vi "Get Spectral Map (U8).vi"(6 "window info":T1={"window type"=10, "window length"=2048} {"window type" items=["None"=0, "Hanning"=1, "Hamming"=2, "Blackman-Harris"=3, "Exact Blackman"=4, "Blackman"=5, "Flat Top"=6, "4 Term B-Harris"=7, "7 Term B-Harris"=8, "Low Sidelobe"=9, "Gaussian"=62]; "window length" min=0}, 7 "dB On (T)":bool=TRUE, 8 "error in (no error)":errorcluster, 9 "type":T4(ring)=enum."RPM-Order", 10 "speed profile":T5 {"speed [RPM]" format="%.2f"; "time [s]" format="%.2f"}, 11 "scaled signal [EU]":waveform(dbl)={"t0"=timestamp(0 s since 1904-01-01), "dt"=0.0, "Y"=[]}) -> (0 "error out":errorcluster, 1 "unit labels":T2, 2 "scales":T3 {"Z scale"."multiplier" format="%.2f"; "Z scale"."offset" format="%.2f"; "Y scale"."multiplier" format="%.2f"; "Y scale"."offset" format="%.2f"; "X scale"."multiplier" format="%.2f"; "X scale"."offset" format="%.2f"}, 3 "spectral map":u8[][](array[numeric]), 4 "actual window":T1={"window type"=10, "window length"=2048} {"window type" items=["None"=0, "Hanning"=1, "Hamming"=2, "Blackman-Harris"=3, "Exact Blackman"=4, "Blackman"=5, "Flat Top"=6, "4 Term B-Harris"=7, "7 Term B-Harris"=8, "Low Sidelobe"=9, "Gaussian"=62]; "window length" min=0})   [LabVIEW 2017]
doc: "Returns the spectral map of <B>scaled signal [EU]</B>. You can use this polymorphic VI to return <B>spectral map</B> as a 2D array of double-precision, floating-point numbers or a 2D array of 8-bit unsigned integers. You must manually select the polymorphic instance to use. Use the DBL instance to obtain more accurate data. Use the U8 instance to reduce memory usage when the VI displays data."
uses:
  <vilib>/addons/Sound and Vibration/Order Analysis/Tach Process/SubVIs/speed profile.ctl
  <vilib>/addons/Sound and Vibration/Order Analysis/Ref Gabor Order Tracking/window information.ctl
  <vilib>/addons/Sound and Vibration/Order Analysis/Ref Gabor Order Tracking/Get Order-RPM Spectral Map (U8).vi
  <vilib>/addons/Sound and Vibration/Order Analysis/Ref Gabor Order Tracking/Get Freq-RPM Spectral Map (U8).vi
  <vilib>/addons/Sound and Vibration/Order Analysis/Ref Gabor Order Tracking/Get Freq-Time Spectral Map (U8).vi
  <vilib>/addons/_NISVFA/_Shared subVIs/Common/svc_Engineering Units to Unit Label.vi
  <vilib>/addons/_NISVFA/_Shared subVIs/Common/svc_Unit Label to Engineering Units.vi
  <vilib>/addons/Sound and Vibration/Order Analysis/Gabor Order Tracking/SoundVib_Gabor.lvlib
  <vilib>/addons/Sound and Vibration/Order Analysis/Tach Process/SoundVib_TachProcess.lvlib
panel:
  # "Get Spectral Map (U8)"
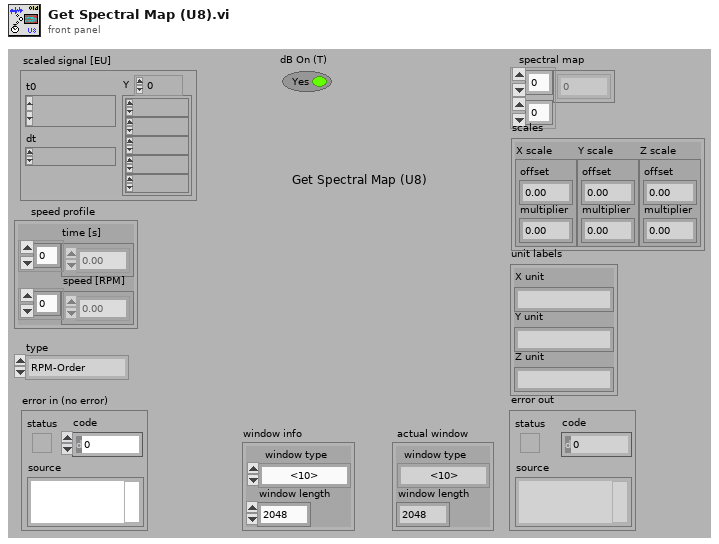
[diagram p1: front panel]
types:
  T1 = typedef "SoundVib_Gabor.lvlib/window information.ctl" = cluster{"window type":u32, "window length":i32}
  T2 = cluster{"X unit":string, "Y unit":string, "Z unit":string}
  T3 = cluster{"X scale":cluster{"offset":dbl, "multiplier":dbl}, "Y scale":cluster{"offset":dbl, "multiplier":dbl}, "Z scale":cluster{"offset":dbl, "multiplier":dbl}}
  T4 = enum16{"Frequency-Time", "Frequency-RPM", "Order-RPM", "RPM-Order"}
  T5 = typedef "SoundVib_TachProcess.lvlib/speed profile.ctl" = cluster{"time [s]":dbl[], "speed [RPM]":dbl[]}
  T6 = typedef "svc_Channel Info.ctl" = cluster{"sensor sensitivity":dbl, "engineering units":T7, "dB reference":dbl, "custom label":string, "weighting filter":T8, "pregain":dbl}
  T7 = typedef "svc_Engineering Units Text Ring.ctl" = u16
  T8 = typedef "svc_Weighting Filter Text Ring.ctl" = u16
  T9 = typedef "SoundVib_Gabor.lvlib/GT RefNum.ctl" = refnum<k1>
  T10 = cluster{"column unit":string, "row unit":string, "unit label":string}
  T11 = cluster{"order scale":cluster{"offset":dbl, "multiplier":dbl}, "rpm scale":cluster{"offset":dbl, "multiplier":dbl}, "quantization info":cluster{"offset":dbl, "multiplier":dbl}}
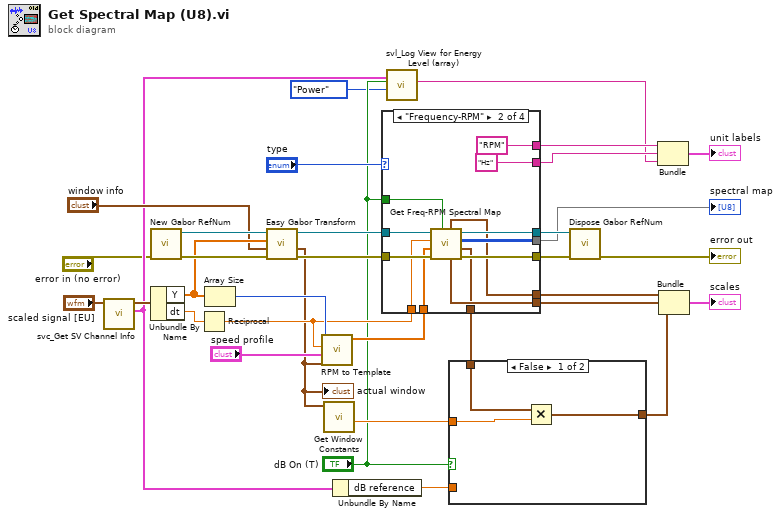
[diagram p0: block diagram]
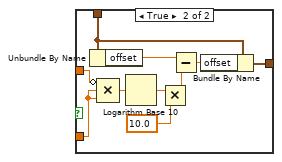
[diagram p2: hidden frame]
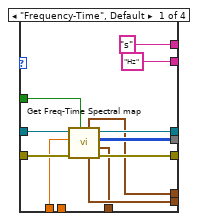
[diagram p3: hidden frame]
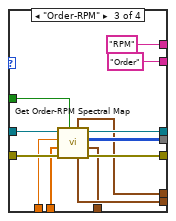
[diagram p4: hidden frame]
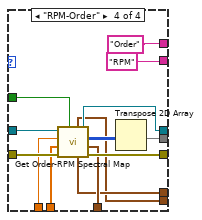
[diagram p5: hidden frame]
diagram:
  n1 = call <vilib>:"svc_Get SV Channel Info.vi"("scaled signal [EU]"="scaled signal [EU]") -> ("channel info"=w3:T6, "dup scaled signal [EU]"=w14:waveform(dbl))  [unwired: 5 in, 4 out]
  n2 = call <vilib>:"New Gabor RefNum.vi"("error in (no error)"="error in (no error)") -> ("error out"=w33:errorcluster, "RefNum"=w34:T9)  [unwired: 8 in]
  n3 = Unbundle By Name(w14) -> ("Y"=w21:dbl[], "dt"=w19:dbl)
  n4 = Reciprocal(x=w19) -> (1/x=w20:dbl)
  n5 = Array Size(array=w21) -> (size(s)=w27:i32)
  n6 = call <vilib>:"Easy Gabor Transform.vi"("error in (no error)"=w33, "window info"="window info", "x[n]"=w21, "RefNum in"=w34) -> ("error out"=w30:errorcluster, "actual window"=w8:T1, "RefNum out"=w31:T9)  [unwired: 3 in, 2 out]
  "actual window" <- w8
  n7 = call <vilib>:"RPM to Template.vi"("window info"=w8, "speed profile"="speed profile", "sampling frequency [Hz]"=w20, "signal length"=w27) -> ("Gabor template"=w25:dbl[])  [unwired: 6 in, 1 out]
  n8 = call <vilib>:"Get Window Constants.vi"("window info"=w8) -> ("multiply factor"=w7:dbl)  [unwired: 9 in, 1 out]
  n9 = Unbundle By Name(w3) -> ("dB reference"=w2:dbl)
  n10 = case shown="\"Frequency-RPM\"" "type" {
    tunnel: [w46 w54 w71 w86] -> w32
    tunnel: w31 -> [w45 w58 w65 w80]
    tunnel: w30 -> [w44 w57 w68 w83]
    tunnel: [w43 w56 w69 w84] -> w29
    tunnel: "dB On (T)" -> [w42 w52 w64 w79]
    tunnel: [w38 w53 w63 w74] -> w13
    tunnel: [w41 w55 w70 w77] -> w9
    tunnel: [w40 w59 w72 w73] -> w12
    tunnel: w20 -> [w39 w50 w66 w81]
    tunnel: w25 -> [_ w51 w67 w82]
    tunnel: ["s" ("row unit") "RPM" ("row unit") "RPM" ("row unit") "Order" ("column unit")] -> w11
    tunnel: ["Hz" ("column unit") "Hz" ("column unit") "Order" ("column unit") "RPM" ("row unit")] -> w10
    tunnel: [w35 w47 w60 w78] -> w17
    frame "Frequency-Time", Default {
      n11 = call-poly <vilib>:"Get Freq-Time Spectral map.vi"("dB On (T)"=w42, "error in (no error)"=w44, "sampling frequency [Hz]"=w39, "RefNum in"=w45) -> ("error out"=w43:errorcluster, "quantization info"=w35:cluster{"offset":dbl, "multiplier":dbl}, "spectral map"=w41:u8[][], "RefNum out"=w46:T9, "frequency scale"=w40:cluster{"offset":dbl, "multiplier":dbl}, "time scale"=w38:cluster{"offset":dbl, "multiplier":dbl})  [unwired: 2 in]
    }
    frame "Frequency-RPM" {
      n12 = call-poly <vilib>:"Get Freq-RPM Spectral Map.vi"("dB On (T)"=w52, "error in (no error)"=w57, "Gabor template"=w51, "sampling frequency [Hz]"=w50, "RefNum in"=w58) -> ("error out"=w56:errorcluster, "quantization info"=w47:cluster{"offset":dbl, "multiplier":dbl}, "spectral map"=w55:u8[][], "RefNum out"=w54:T9, "frequency scale"=w59:cluster{"offset":dbl, "multiplier":dbl}, "rpm scale"=w53:cluster{"offset":dbl, "multiplier":dbl})  [unwired: 1 in]
    }
    frame "Order-RPM" {
      n13 = call-poly <vilib>:"Get Order-RPM Spectral Map.vi"("dB On (T)"=w64, "error in (no error)"=w68, "Gabor template"=w67, "sampling frequency [Hz]"=w66, "RefNum in"=w65) -> ("error out"=w69:errorcluster, "quantization info"=w60:cluster{"offset":dbl, "multiplier":dbl}, "spectral map"=w70:u8[][], "RefNum out"=w71:T9, "order scale"=w72:cluster{"offset":dbl, "multiplier":dbl}, "rpm scale"=w63:cluster{"offset":dbl, "multiplier":dbl})  [unwired: 1 in]
    }
    frame "RPM-Order" {
      n14 = call-poly <vilib>:"Get Order-RPM Spectral Map.vi"("dB On (T)"=w79, "error in (no error)"=w83, "Gabor template"=w82, "sampling frequency [Hz]"=w81, "RefNum in"=w80) -> ("error out"=w84:errorcluster, "quantization info"=w78:cluster{"offset":dbl, "multiplier":dbl}, "spectral map"=w85:u8[][], "RefNum out"=w86:T9, "order scale"=w74:cluster{"offset":dbl, "multiplier":dbl}, "rpm scale"=w73:cluster{"offset":dbl, "multiplier":dbl})  [unwired: 1 in]
      n15 = Transpose 2D Array(2D array=w85) -> (transposed array=w77:u8[][])
    }
  }
  "spectral map" <- w9
  n16 = call <vilib>:"svl_Log View for Energy Level (array).vi"("channel info"=w3, "view mode"=enum16{"Power", "Amplitude"}."Power", "dB On (T)"="dB On (T)") -> ("unit label"=w4:string)  [unwired: 6 in, 2 out]
  n17 = case shown="False" "dB On (T)" {
    tunnel: [w87 w93] -> w16
    tunnel: w17 -> [w89 w96]
    tunnel: w7 -> [w88 w92]
    tunnel: w2 -> [_ w90]
    frame False {
      n18 = Multiply(x=w89, y=w88) -> (x*y=w87:cluster{"offset":dbl, "multiplier":dbl})
    }
    frame True {
      n19 = Unbundle By Name(w96) -> ("offset"=w94:dbl)
      n20 = Compound Arithmetic op=MULTIPLY(invert w92, w90, w90) -> (w91:dbl)
      n21 = Logarithm Base 10(1:w91) -> (0:w98:dbl)
      n22 = Multiply(x=w98, y=10.0) -> (x*y=w97:dbl)
      n23 = Subtract(x=w94, y=w97) -> (x-y=w95:dbl)
      n24 = Bundle By Name(cluster=w96, "offset"=w95) -> (w93:cluster{"offset":dbl, "multiplier":dbl})
    }
  }
  n25 = call <vilib>:"Dispose Gabor RefNum.vi"("error in (no error)"=w29, "RefNum in"=w32) -> ("error out"=→"error out":errorcluster)  [unwired: 6 in]
  n26 = Bundle("column unit"=w11, "row unit"=w10, "unit label"=w4) -> (→"unit labels":T10)  [unwired: 1 in]
  n27 = Bundle("order scale"=w13, "rpm scale"=w12, "quantization info"=w16) -> (→"scales":T11)  [unwired: 1 in]
